vi "Annouce.vi"(5 "port or service name":u16=50001, 7 "Address":string="255.255.255.255", 8 "error in (no error)":errorcluster, 9 "Command Queue":refnum<class "Message Enqueuer.lvclass">, 10 "String":string="FLATXML", 11 "Receiver in":refnum<class "Receiver.lvclass">) -> (0 "error out":errorcluster, 3 "Receiver out":refnum<class "Receiver.lvclass">)   [LabVIEW 2013, in "Receiver.lvlib" / "Receiver.lvclass"]
uses:
  Receiver.lvclass
  <vilib>/ActorFramework/Message Enqueuer/Message Enqueuer.lvclass
  <vilib>/ActorFramework/Actor/Actor.lvclass/Actor.ctl
  <vilib>/ActorFramework/Message Enqueuer/Message Enqueuer.lvclass/Message Enqueuer.ctl
  Receiver.lvclass/Receiver.ctl
  Receiver Messages/Listen Msg/Listen Msg.lvclass/Listen Msg.ctl
  <vilib>/ActorFramework/Message Enqueuer/Init from Existing Queue.vi
  <vilib>/ActorFramework/Message Enqueuer/Enqueue.vi
  <vilib>/ActorFramework/Message Priority Queue/Priority Enqueue.vi
  Receiver Messages/Listen Msg/Listen Msg.lvclass
  <vilib>/ActorFramework/Actor/Actor.lvclass
panel:
  out "error out 2":errorcluster
  in  "timeout ms (25000)":i32=25
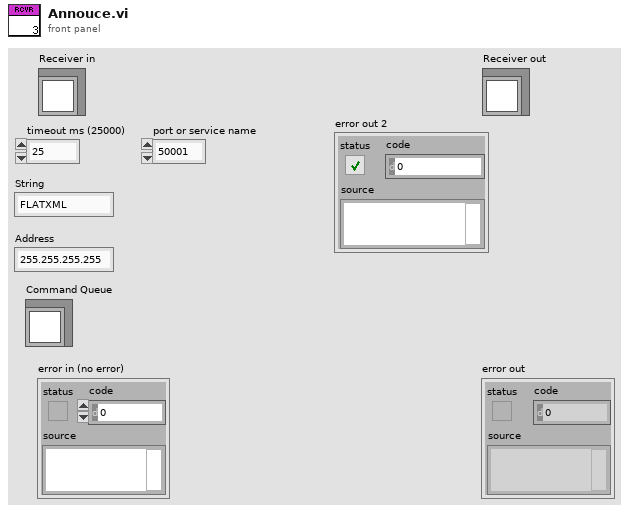
[diagram p1: front panel]
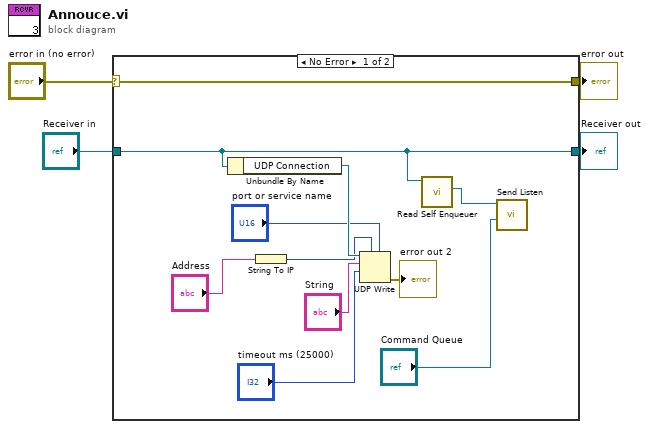
[diagram p0: block diagram]
diagram:
  n1 = case shown="No Error" "error in (no error)" {
    selector: "error in (no error)" -> [w9 w17]
    tunnel: [w9 w17] -> w3
    tunnel: [w7 w16] -> w1
    tunnel: "Receiver in" -> [w7 w16]
    frame No Error {
      n2 = Unbundle By Name(w7) -> ("UDP Connection"=w15:refnum<k16>)
      n3 = String To IP(1:"Address") -> (0:w13:u32)
      n4 = UDP Write(address=w13, port or service name="port or service name", connection ID=w15, data in="String", 9:"timeout ms (25000)") -> (error out=→"error out 2":errorcluster)  [unwired: 1 in, 1 out]
      n5 = call <vilib>:"Read Self Enqueuer.vi"("Actor"=w7) -> ("Self Enqueuer"=w6:refnum<class "Message Enqueuer.lvclass">)  [unwired: 10 in]
      n6 = call "Send Listen.vi"("Command Queue"="Command Queue", "Message Enqueuer"=w6) -> ()  [unwired: 8 in, 2 out]
    }
    frame Error {
    }
  }
  "error out" <- w3
  "Receiver out" <- w1
